vi "模拟电容电压.vi"(5 "Vmax":dbl, 6 "C":dbl, 7 "R":dbl) -> (0 "当前电压":dbl)   [LabVIEW 2024]
panel:
  in  "放电":bool
  in  "充电":bool
  out "充电状态显示":string
  in  "退出":bool
  in  "暂停":bool
  out "波形图表":dbl(graph)
  # "使用说明\\\\\n1、使用前设置电容的电阻R、电容C、最大电压Vmax\n2、切换充电与放电状态，需要先点击暂停按钮再进行切换\n3、先复位已按下的按钮，再去按其他按钮"
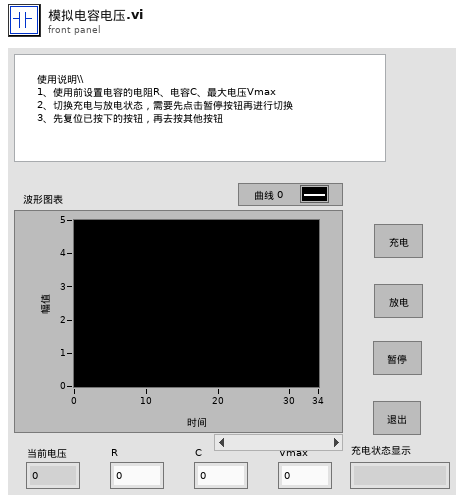
[diagram p1: front panel]
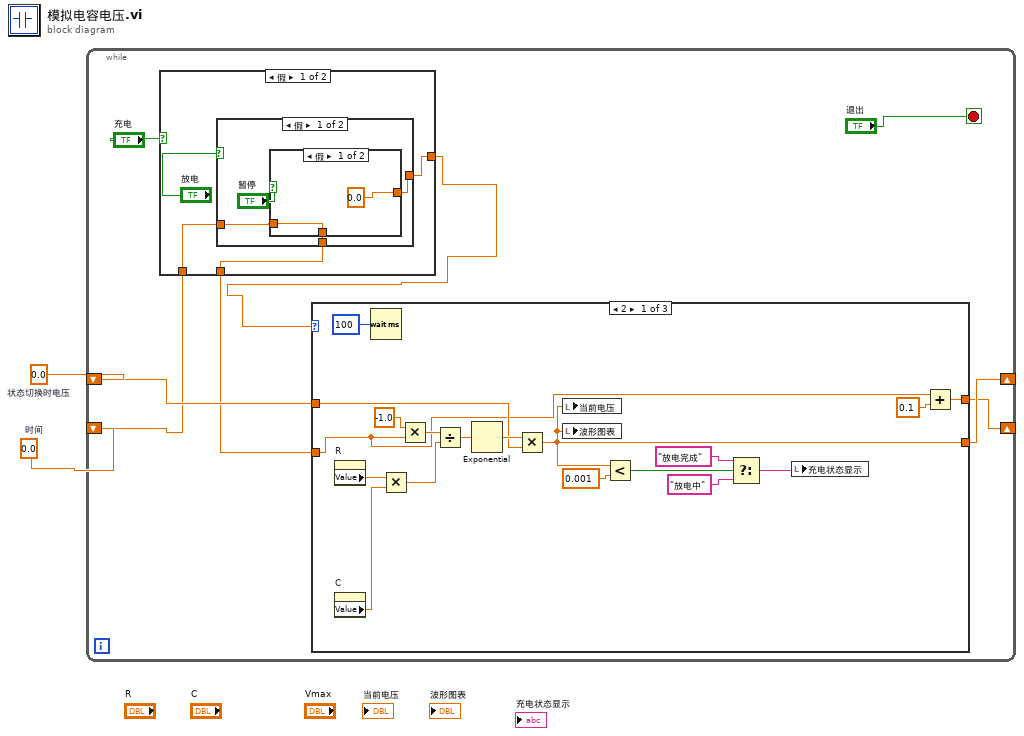
[diagram p0: block diagram]
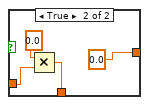
[diagram p2: hidden frame]
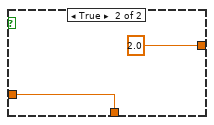
[diagram p3: hidden frame]
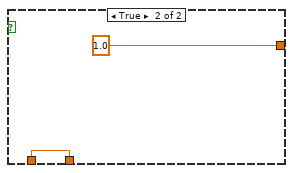
[diagram p4: hidden frame]
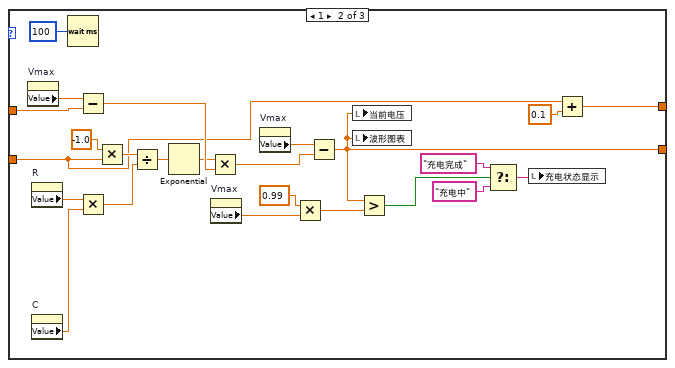
[diagram p5: hidden frame]
diagram:
  w1 = 0.0  # 时间
  w2 = 0.0  # 状态切换时电压
  n1 = while {
    shift-right: [w8] -> _
    shift-left: w1 -> [w3]
    shift-right: [w9] -> _
    shift-left: w2 -> [w10]
    stop <- "退出" stop-if-true
    n2 = case shown="假" "充电" {
      tunnel: [w14 1.0] -> w6
      tunnel: [w12 w27] -> w4
      tunnel: w3 -> [w11 w27]
      frame False {
        n3 = case shown="假" "放电" {
          tunnel: [w18 2.0] -> w14
          tunnel: [w16 w25] -> w12
          tunnel: w11 -> [w15 w25]
          frame False {
            n4 = case shown="假" "暂停" {
              tunnel: [0.0 0.0] -> w18
              tunnel: [w19 w23] -> w16
              tunnel: w15 -> [w19 w22]
              frame False {
              }
              frame True {
                n5 = Multiply(x=0.0, y=w22) -> (x*y=w23:dbl)
              }
            }
          }
          frame True {
          }
        }
      }
      frame True {
      }
    }
    n6 = case shown="2" w6 {
      tunnel: w10 -> [w30 w52 w72]
      tunnel: [w32 w49 w71] -> w8
      tunnel: [w31 w48 w72] -> w9
      tunnel: w4 -> [w29 w47 w71]
      frame 2 {
        n7 = property on="R" class="DigNum (严格)"() -> ("Value"=w43:dbl)  [unwired: 2 in, 2 out]
        n8 = property on="C" class="DigNum (严格)"() -> ("Value"=w44:dbl)  [unwired: 2 in, 2 out]
        n9 = Wait (ms)(milliseconds to wait=u32 100 ("等待时间（毫秒）")) -> ()  [unwired: 1 out]
        n10 = Multiply(x=w43, y=w44) -> (x*y=w40:dbl)
        n11 = Multiply(x=-1.0, y=w29) -> (x*y=w41:dbl)
        n12 = Divide(x=w41, y=w40) -> (x/y=w39:dbl)
        n13 = Exponential(1:w39) -> (0:w42:dbl)
        n14 = Multiply(x=w42, y=w30) -> (x*y=w31:dbl)
        n15 = local write "当前电压"(w31) -> ()
        n16 = local write "波形图表"(w31) -> ()
        n17 = Less?(x=w31, y=0.001) -> (x < y?=w45:bool)
        n18 = Select(t="放电完成", s=w45, f="放电中") -> (s? t:f=w46:string)
        n19 = local write "充电状态显示"(w46) -> ()
        n20 = Add(x=w29, y=0.1) -> (x+y=w32:dbl)
      }
      frame 1 {
        n21 = property on="Vmax" class="DigNum (严格)"() -> ("Value"=w65:dbl)  [unwired: 2 in, 2 out]
        n22 = property on="R" class="DigNum (严格)"() -> ("Value"=w60:dbl)  [unwired: 2 in, 2 out]
        n23 = property on="C" class="DigNum (严格)"() -> ("Value"=w61:dbl)  [unwired: 2 in, 2 out]
        n24 = Wait (ms)(milliseconds to wait=u32 100 ("等待时间（毫秒）")) -> ()  [unwired: 1 out]
        n25 = Subtract(x=w65, y=w52) -> (x-y=w66:dbl)
        n26 = Multiply(x=w60, y=w61) -> (x*y=w58:dbl)
        n27 = Multiply(x=-1.0, y=w47) -> (x*y=w59:dbl)
        n28 = Divide(x=w59, y=w58) -> (x/y=w57:dbl)
        n29 = Exponential(1:w57) -> (0:w64:dbl)
        n30 = Multiply(x=w64, y=w66) -> (x*y=w68:dbl)
        n31 = property on="Vmax" class="DigNum (严格)"() -> ("Value"=w62:dbl)  [unwired: 2 in, 2 out]
        n32 = property on="Vmax" class="DigNum (严格)"() -> ("Value"=w67:dbl)  [unwired: 2 in, 2 out]
        n33 = Multiply(x=0.99, y=w62) -> (x*y=w63:dbl)
        n34 = Subtract(x=w67, y=w68) -> (x-y=w48:dbl)
        n35 = local write "当前电压"(w48) -> ()
        n36 = local write "波形图表"(w48) -> ()
        n37 = Greater?(x=w48, y=w63) -> (0:w70:bool)
        n38 = Select(t="充电完成", s=w70, f="充电中") -> (s? t:f=w69:string)
        n39 = local write "充电状态显示"(w69) -> ()
        n40 = Add(x=w47, y=0.1) -> (x+y=w49:dbl)
      }
      frame 0, Default {
      }
    }
  }
